vi "Generate Paths.vi"(10 "Number of Paths":i32, 11 "Array":i32[][](array[numeric])) -> (3 "Paths":T1[][](array[typedef]))   [LabVIEW 2019, in "Day 15.lvlib"]
uses:
  Day 15.lvlib
  Day 11/Controls/Side.ctl
  <vilib>/numeric/Random Number (Range) U64.vi
  <vilib>/numeric/sub_Random U32.vi
  Day 11/Day 11.lvlib
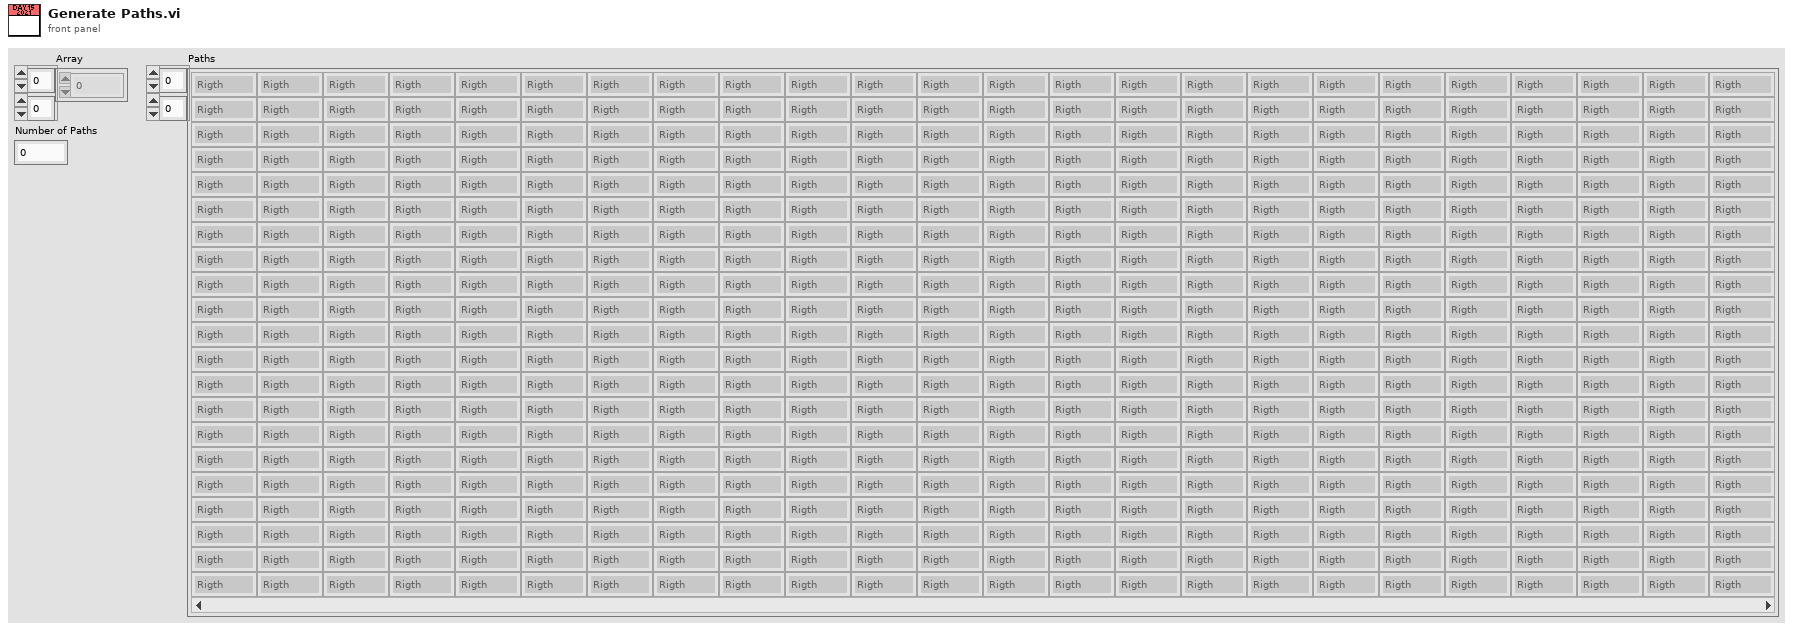
[diagram p1: front panel]
types:
  T1 = typedef "Day 11.lvlib/Side.ctl" = enum16{"Rigth", "Left", "Down", "Up", "Rigth Up", "Rigth Down", "Left Up", "Left Down"}
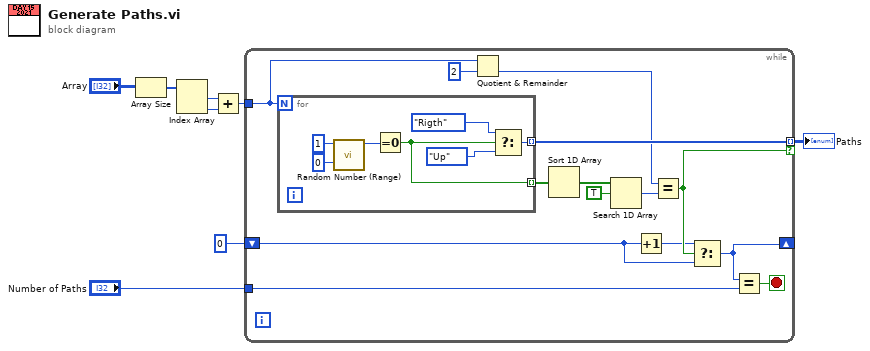
[diagram p0: block diagram]
diagram:
  n1 = Array Size(array="Array") -> (size(s)=w7:i32[])
  n2 = Index Array(array=w7) -> (element #1=w5:i32, element #2=w6:i32)  [unwired: 2 in]
  n3 = Add(x=w5, y=w6) -> (x+y=w3:i32)
  n4 = while {
    tunnel: [w22] -> w4 mode=indexing if=w14
    tunnel: w3 -> [w19]
    shift-right: [w11] -> _
    shift-left: 0 ("y") -> [w12]
    tunnel: "Number of Paths" -> [w10]
    stop <- w9 stop-if-true
    n5 = for {
      N: w19 -> [_]
      tunnel: [w27] -> w22 mode=indexing
      tunnel: [w23] -> w21 mode=indexing
      n6 = call-poly <vilib>:"Random Number (Range).vi"("lower bound (0)"=u64 0, "upper bound (100)"=u64 1) -> ("number"=w24:u64)  [unwired: 9 in]
      n7 = Equal To 0?(x=w24) -> (x = 0?=w23:bool)
      n8 = Select(t=Side."Rigth" ("Side"), s=w23, f=Side."Up" ("Side")) -> (s? t:f=w27:T1)
    }
    n9 = Quotient & Remainder(x=w19, y=2) -> (floor(x/y)=w18:i32)  [unwired: 1 out]
    n10 = Sort 1D Array(array=w21) -> (sorted array=w17:bool[])
    n11 = Search 1D Array(1D array=w17, element=TRUE) -> (index of element=w15:i32)  [unwired: 1 in]
    n12 = Increment(x=w12) -> (x+1=w13:i32)
    n13 = Equal?(x=w18, y=w15) -> (x = y?=w14:bool)
    n14 = Select(t=w13, s=w14, f=w12) -> (s? t:f=w11:i32)
    n15 = Equal?(x=w11, y=w10) -> (x = y?=w9:bool)
  }
  "Paths" <- w4
